vi "Configure Input Filter.vi"(0 "VISA resource name":refnum<visa-resource-name>, 1 "Enable Filter (F: Off)":bool, 5 "Input (0:A)":u16(ring) items=["A", "B", "C", "D"], 7 "Filter Points (8)":dbl=8.0, 9 "Filter Window (1 %)":dbl=1.0, 11 "error in (no error)":errorcluster) -> (4 "VISA resource name out":refnum<visa-resource-name>, 15 "error out":errorcluster)   [LabVIEW 2019, in "Lake Shore 336.lvlib"]
doc: "This VI configures the sensor input filter. The filter applies exponential smoothing to the sensor input readings. If the filter is turned on for a sensor input, all reading values for that input are filtered. The filter is a running average so it does not change the update rate of an input. Filtered readings are used for displayed readings only, not for control functions."
uses:
  Lake Shore 336.lvlib
  Instance           1 30Saved   Configure Input Filter .vi
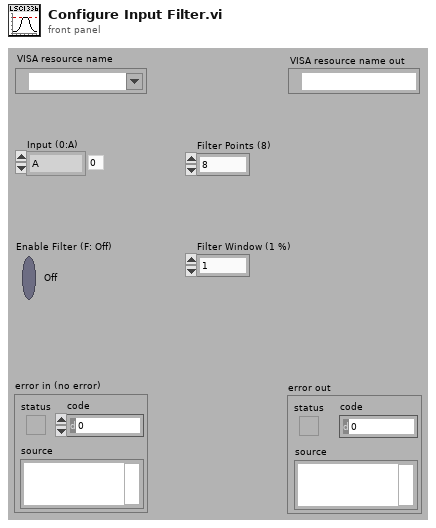
[diagram p1: front panel]
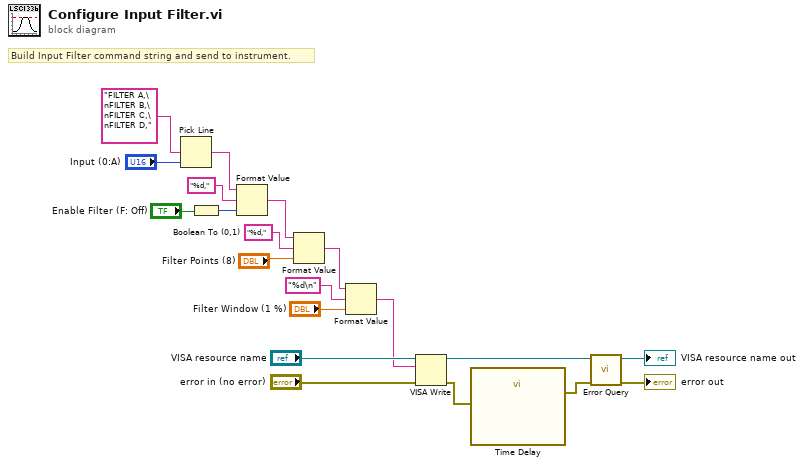
[diagram p0: block diagram]
diagram:
  # "Build Input Filter command string and send to instrument."
  n1 = Pick Line(multi-line string="FILTER A,\nFILTER B,\nFILTER C,\nFILTER D,", line index="Input (0:A)") -> (output string=w11:string)  [unwired: 1 in]
  n2 = Boolean To (0,1)(Boolean="Enable Filter (F: Off)") -> (0, 1=w12:i16)
  n3 = Format Value(string ("")=w11, format string="%d,", value (0)=w12) -> (output string=w9:string)
  n4 = Format Value(string ("")=w9, format string="%d,", value (0)="Filter Points (8)") -> (output string=w8:string)
  n5 = Format Value(string ("")=w8, format string="%d\n", value (0)="Filter Window (1 %)") -> (output string=w1:string)
  n6 = VISA Write(VISA resource name="VISA resource name", write buffer=w1, error in (no error)="error in (no error)") -> (VISA resource name out=w18:refnum<visa-resource-name>, error out=w5:errorcluster)  [unwired: 1 out]
  n7 = call "Time Delay"("error in (no error)"=w5) -> ("error out"=w4:errorcluster)  [unwired: 10 in]
  n8 = call "Error Query.vi"("error in (no error)"=w4, "VISA resource name"=w18) -> ("error out"=→"error out":errorcluster, "VISA resource name out"=→"VISA resource name out":refnum<visa-resource-name>)  [unwired: 7 in, 1 out]
